vi "UI Build Do CMD.vi"(8 "error in (no error)":errorcluster, 9 "Message Data":variant, 11 "DAQ DO ON-OFF":refnum<queue>) -> (0 "error out":errorcluster, 1 "CMD Data":variant, 3 "CMD Queue out":refnum<queue>)   [LabVIEW 2020]
uses:
  support/Message Queue/Message Cluster.ctl
  support/Message Queue/Message Queue.lvlib
panel:
  in  "Registers":T1(ring)=enum."FixElevationValve"
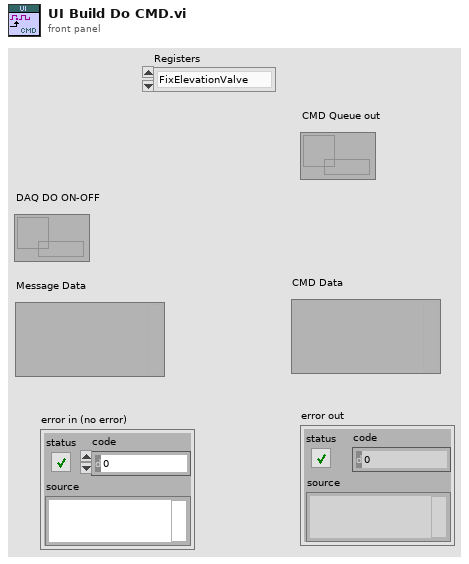
[diagram p1: front panel]
types:
  T1 = enum16{"FixActuatorsValve", "FixElevationValve", "FixInsulationValve", "LoadSenseValve", "LoadModeValve", "Chiller24V", "SuctionValve_OpenCMD ", "SuctionValve_CloseCMD ", "ChillerValve", "EnableAirPressureValve ", "MainMotor", "MotorFan", "MotorHeatExchange", "EnablePressure", "StartHeating", "StartCommand"}
  T2 = cluster{"Channel":enum16{"FixActuatorsValve", "FixElevationValve", "FixInsulationValve", "LoadSenseValve", "LoadModeValve", "Chiller24V", "SuctionValve_OpenCMD ", "SuctionValve_CloseCMD ", "ChillerValve", "EnableAirPressureValve ", "MainMotor", "MotorFan", "MotorHeatExchange", "EnablePressure", "StartHeating", "StartCommand"}, "Status":bool}
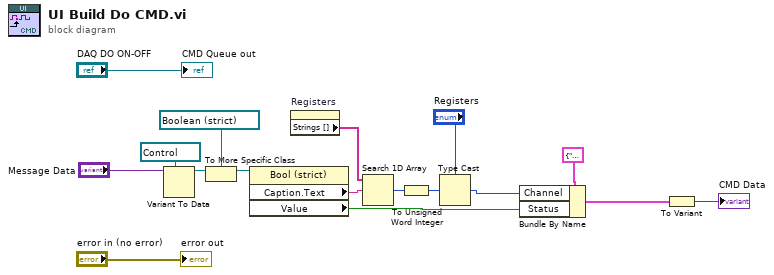
[diagram p0: block diagram]
diagram:
  n1 = Variant To Data(type=refnum<vi> refnum ("CtlRef"), Variant="Message Data") -> (data=w7:refnum<vi>)  [unwired: 1 in, 1 out]
  n2 = To More Specific Class(target class=refnum<vi> refnum ("CV_In_03"), reference=w7) -> (specific class reference=w4:refnum<vi>)  [unwired: 1 in, 1 out]
  n3 = property class="Bool (strict)"(reference=w4) -> ("Caption.Text"=w11:string, "Value"=w15:bool)  [unwired: 1 in, 2 out]
  n4 = property on="Registers" class="Enum (strict)"() -> ("Strings []"=w10:string[])  [unwired: 2 in, 2 out]
  n5 = Search 1D Array(1D array=w10, element=w11) -> (index of element=w8:i32)  [unwired: 1 in]
  n6 = To Unsigned Word Integer(number=w8) -> (unsigned 16bit integer=w9:u16)
  n7 = Type Cast(type="Registers", x=w9) -> (*(type *) &x=w16:T1)
  n8 = Bundle By Name(cluster=T2 {"Channel"=enum."FixElevationValve", "Status"=FALSE}, "Channel"=w16, "Status"=w15) -> (w17:T2)
  n9 = To Variant(anything=w17) -> (Variant=→"CMD Data":variant)
  "CMD Queue out" <- "DAQ DO ON-OFF"
  "error out" <- "error in (no error)"
